vi "Do.vi"(8 "error in (no error)":errorcluster, 10 "Actor in":refnum<class "Actor.lvclass">, 11 "View Front Panel Msg":refnum<class "View Front Panel Msg.lvclass">) -> (0 "error out":errorcluster, 2 "Actor out":refnum<class "Actor.lvclass">)   [LabVIEW 2013, in "PluginInterface.lvlib" / "View Front Panel Msg.lvclass"]
uses:
  View Front Panel Msg.lvclass
  Actor Framework.lvlibp/Actor/Actor.lvclass
  PluginInterface.lvclass
  View Front Panel Msg.lvclass/View Front Panel Msg.ctl
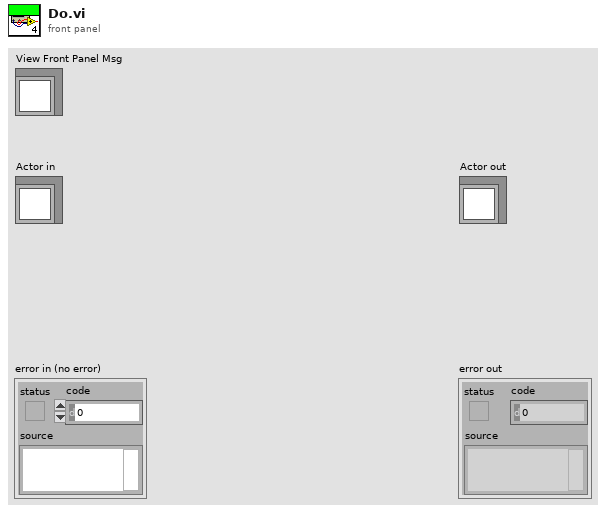
[diagram p1: front panel]
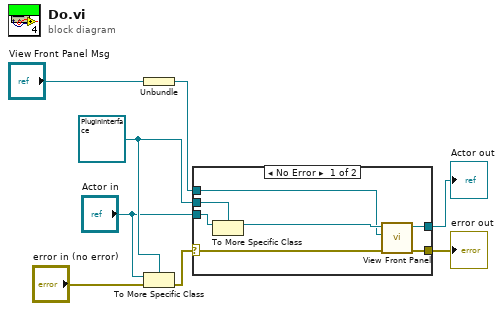
[diagram p0: block diagram]
diagram:
  w4 = refnum<class "PluginInterface.lvclass"> refnum ("PluginInterface.lvlib:PluginInterface.lvclass")
  n1 = Unbundle("View Front Panel Msg") -> (w7:refnum<vi>)
  n2 = To More Specific Class(target class=w4, reference="Actor in", error in="error in (no error)") -> (error out=w8:errorcluster)  [unwired: 1 out]
  n3 = case shown="No Error" w8 {
    selector: w8 -> [w11 w17]
    tunnel: [w13 w17] -> w2
    tunnel: [w12 w16] -> w1
    tunnel: "Actor in" -> [w15 w16]
    tunnel: w4 -> [w14 _]
    tunnel: w7 -> [w9 _]
    frame No Error {
      n4 = To More Specific Class(target class=w14, reference=w15) -> (specific class reference=w10:refnum<class "PluginInterface.lvclass">)  [unwired: 1 in, 1 out]
      n5 = call-dynamic "View Front Panel.vi"("error in (no error)"=w11, "SubPnl Refnum"=w9, "PluginInterface in"=w10) -> ("error out"=w13:errorcluster, "PluginInterface out"=w12:refnum<class "PluginInterface.lvclass">)  [unwired: 7 in]
    }
    frame Error {
      # "If type check fails, pass the original object out again."
    }
  }
  "error out" <- w2
  "Actor out" <- w1
